vi "GaGe_TrigConfigAll.vi"(4 "Trigger":T2 {"Slope" items=["Positive", "Negative"]; "Level" format="%.2f"; "Coupling" items=["DC 1 MOhm", "AC 1 MOhm", "HF Reject", "LF Reject", "AC Plus HF Reject"]; "Source" items=["Chan 1", "External"]}, 5 "Handle Cluster":T1) -> (2 "Handle Cluster Out":T1)   [LabVIEW 2022 SP3]
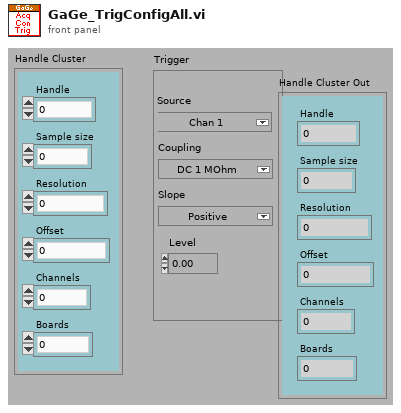
[diagram p1: front panel]
types:
  T1 = cluster{"Handle":u32, "Sample size":u32, "Resolution":i32, "Offset":i32, "Channels":u32, "Boards":u32}
  T2 = cluster{"Source":u16, "Coupling":u16, "Slope":u16, "Level":dbl}
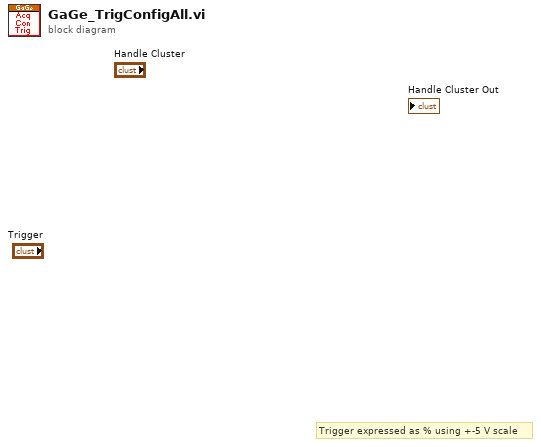
[diagram p0: block diagram]
diagram:
  # "Trigger expressed as % using +-5 V scale"
